vi "Call.vi"(7 "Actor in":refnum<class "Actor.lvclass">, 9 "From Msg Event":bool, 10 "Msg":refnum<class "Msg.lvclass">) -> (0 "Error out":errorcluster, 2 "Msg Output":refnum<class "Msg Output.lvclass">, 5 "Actor out":refnum<class "Actor.lvclass">)   [LabVIEW 2025, in "jettl.lvlib" / "Actor.lvlib"]
uses:
  Actor.lvlib
  Actor/Actor.lvclass
  Msg/Msg.lvclass
  Msg Output/Msg Output.lvclass
  Attributes/Attributes/Attributes.lvclass
  Error/Error.lvlib
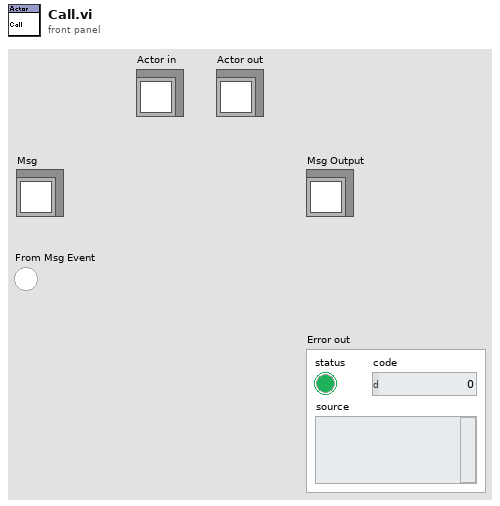
[diagram p1: front panel]
types:
  T1 = typedef "jettl.lvlib/Actor.lvlib/Msg Set.ctl" = set{refnum<class "Msg.lvclass">}
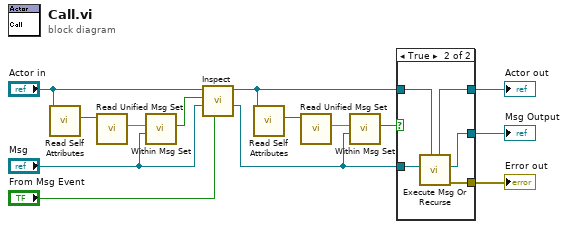
[diagram p0: block diagram]
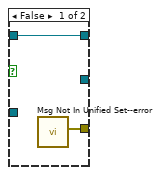
[diagram p2: hidden frame]
diagram:
  n1 = call-dynamic "Read Self Attributes.vi"("Actor in"="Actor in") -> ("Self Attributes"=w14:refnum<class "Attributes.lvclass">)  [unwired: 10 in]
  n2 = call-dynamic "Read Unified Msg Set.vi"("Attributes in"=w14) -> ("Unified Msg Set"=w13:T1)  [unwired: 10 in]
  n3 = call "Within Msg Set.vi"("Msg"="Msg", "Msg Set"=w13) -> ("Within Msg Set"=w12:bool)  [unwired: 9 in]
  n4 = call-dynamic "Inspect.vi"("From Msg Event"="From Msg Event", "Msg in"="Msg", "Within Msg Set"=w12, "Actor in"="Actor in") -> ("Msg out"=w3:refnum<class "Msg.lvclass">, "Actor out"=w4:refnum<class "Actor.lvclass">)  [unwired: 6 in]
  n5 = call-dynamic "Read Self Attributes.vi"("Actor in"=w4) -> ("Self Attributes"=w6:refnum<class "Attributes.lvclass">)  [unwired: 10 in]
  n6 = call-dynamic "Read Unified Msg Set.vi"("Attributes in"=w6) -> ("Unified Msg Set"=w5:T1)  [unwired: 10 in]
  n7 = call "Within Msg Set.vi"("Msg"=w3, "Msg Set"=w5) -> ("Within Msg Set"=w2:bool)  [unwired: 9 in]
  n8 = case shown="True" w2 {
    tunnel: w4 -> [w16 w21]
    tunnel: [w16 w20] -> w9
    tunnel: w3 -> [_ w18]
    tunnel: [w15 w19] -> w8
    tunnel: [_ w17] -> w1
    frame False {
      n9 = call "Msg Not In Unified Set--error.vi"() -> ("Error"=w15:errorcluster)  [unwired: 11 in]
    }
    frame True {
      n10 = call "Execute Msg Or Recurse.vi"("Actor in"=w21, "Msg"=w18) -> ("Error out"=w19:errorcluster, "Msg Output"=w17:refnum<class "Msg Output.lvclass">, "Actor out"=w20:refnum<class "Actor.lvclass">)  [unwired: 7 in]
    }
  }
  "Actor out" <- w9
  "Error out" <- w8
  "Msg Output" <- w1
